vi "Initialize.vi"(8 "error in (no error)":errorcluster, 10 "DeviceName":string, 11 "DG645 in":refnum<class "SMC100.lvclass">) -> (0 "error out":errorcluster, 1 "new command(s)":string, 2 "DeviceName":string, 3 "DG645 out":refnum<class "SMC100.lvclass">)   [LabVIEW 2020, in "SMC100.lvclass"]
uses:
  SMC100.lvclass
  SMC100.lvclass/SMC100.ctl
  source/Device Drivers/BaseDriver/BaseDriver.lvclass
panel:
  out "Devicetype\nvariable list":string[][](array[string])
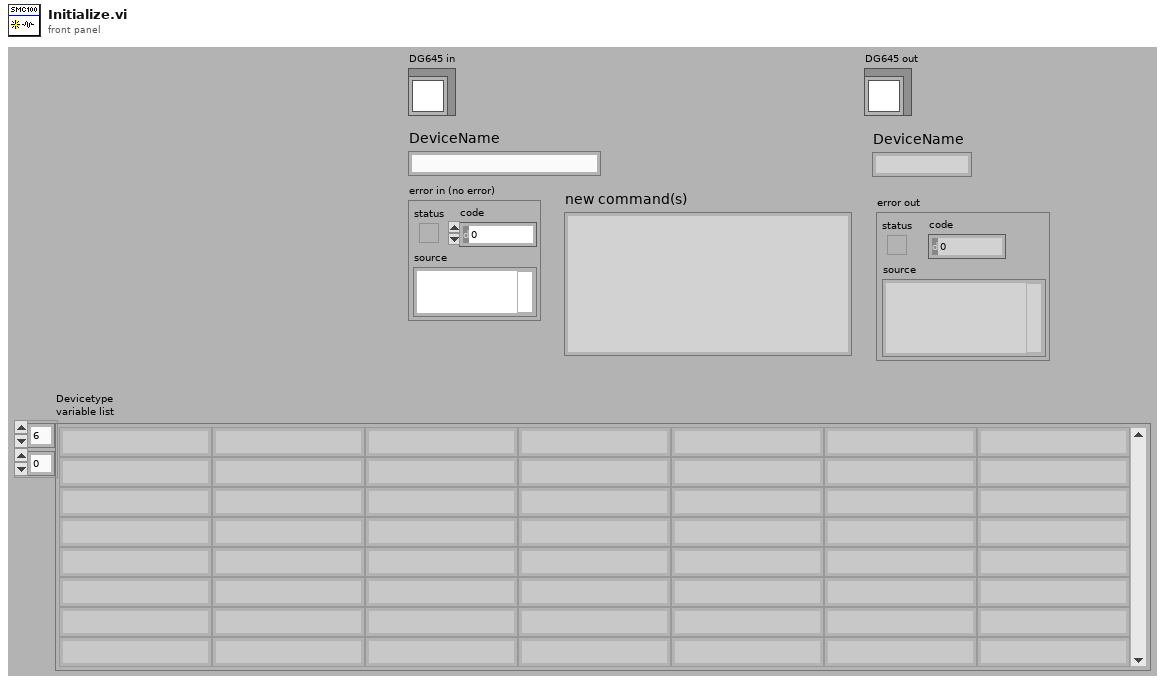
[diagram p1: front panel]
types:
  T1 = typedef "SMC100.lvclass/settingsDG645_TypDef.ctl" = cluster{"timeout":T2, "ControllerAddress":dbl, "VisaResourceName":string, "DeviceName":string, "Position":T2, "Name":string, "Home":T3, "Offset":T2}
  T2 = typedef "BaseDriver.lvclass/numericVariable_TypeDef.ctl" = cluster{"Value":dbl, "Min":dbl, "Max":dbl, "StepSize":dbl, "Tolerance":dbl, "ValueActual":dbl}
  T3 = typedef "OnOffTypeDef.ctl" = enum16{"off", "on"}
  T4 = cluster{"VISA resource name":refnum<visa-resource-name>, "Device name":string, "Controller address":i32, "error":errorcluster}
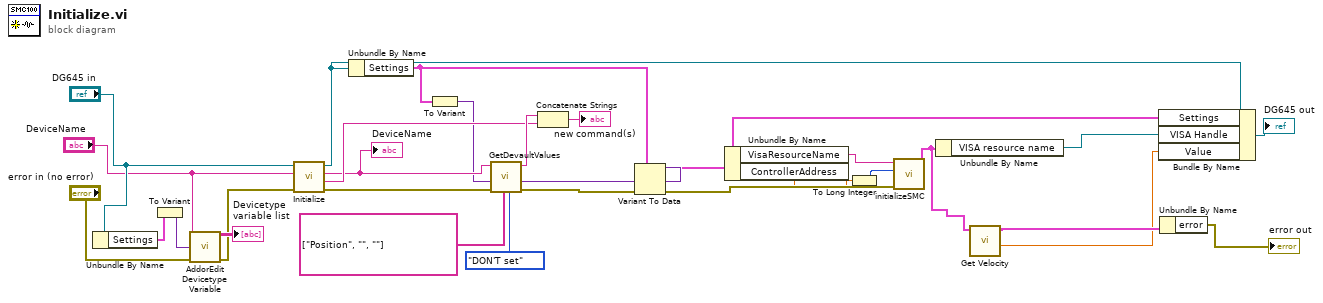
[diagram p0: block diagram]
diagram:
  n1 = Unbundle By Name("DG645 in") -> ("Settings"=w9:T1)
  n2 = To Variant(anything=w9) -> (Variant=w8:variant)
  n3 = call "AddorEdit Devicetype Variable.vi"("Device Name"="DeviceName", "Settings variant"=w8, "error in"="error in (no error)") -> ("Devicetype variable list"=→"Devicetype\nvariable list":string[][], "error out"=w6:errorcluster)  [unwired: 11 in]
  n4 = call-parent "Initialize.vi"("error in (no error)"=w6, "DeviceName"="DeviceName", "BaseDriver in"="DG645 in") -> ("error out"=w24:errorcluster, "new command(s)"=w28:string, "DeviceName"=w22:string, "BaseDriver out"=w27:refnum<class "SMC100.lvclass">)  [unwired: 5 in]
  "DeviceName" <- w22
  n5 = Unbundle By Name(w27) -> ("Settings"=w20:T1)
  n6 = To Variant(anything=w20) -> (Variant=w21:variant)
  n7 = call "GetDevaultValues.vi"("set or DON'T set"=enum16{"set", "DON'T set"}."DON'T set", "set following Variables (empty = all avriables)"=string[] ["Position", "", ""], "error in (no error)"=w24, "variant"=w21, "Device Name"=w22) -> ("error out"=w23:errorcluster, "variant out"=w29:variant, "new command(s)"=w30:string)  [unwired: 4 in]
  n8 = Concatenate Strings(w30, w28) -> (→"new command(s)":string)
  n9 = Variant To Data(error in=w23, type=w20, Variant=w29) -> (data=w19:T1, error out=w15:errorcluster)
  n10 = Unbundle By Name(w19) -> ("VisaResourceName"=w16:string, "ControllerAddress"=w13:dbl)
  n11 = To Long Integer(number=w13) -> (32bit integer=w12:i32)
  n12 = call "initializeSMC.vi"("error in (no error)"=w15, "Controller address"=w12, "VisaRresourceName"=w16) -> ("Device Connection Cluster"=w3:T4)  [unwired: 8 in]
  n13 = Unbundle By Name(w3) -> ("VISA resource name"=w14:refnum<visa-resource-name>)
  n14 = call "Get Velocity.vi"("Connection Cluster in"=w3) -> ("Velocity"=w1:dbl, "Connection Cluster out"=w2:T4)  [unwired: 8 in, 1 out]
  n15 = Bundle By Name(cluster=w27, "Settings"=w19, "VISA Handle"=w14, "Value"=w1) -> (→"DG645 out":refnum<class "SMC100.lvclass">)
  n16 = Unbundle By Name(w2) -> ("error"=→"error out":errorcluster)
